vi "SendMsg.vi"(8 "error in (no error)":errorcluster, 11 "DataIn":T1={"MsgPageSelect"=enum."Action", "LogType"=enum."Manual", "Msg"="", "Time"=""}) -> (0 "error out":errorcluster)   [LabVIEW 2019, in "MsgShowAndLog.lvlib"]
uses:
  MsgShowAndLog.lvlib
  Ctrl/MsgDataInput.ctl
  Ctrl/MsgPageSelect.ctl
  Ctrl/LogType.ctl
  global/MsgQue.vi
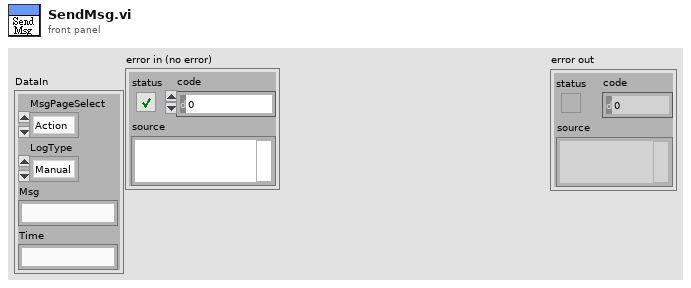
[diagram p1: front panel]
types:
  T1 = typedef "MsgDataInput.ctl" = cluster{"MsgPageSelect":T2, "LogType":T3, "Msg":string, "Time":string}
  T2 = typedef "MsgShowAndLog.lvlib/MsgPageSelect.ctl" = enum16{"System", "Comm", "IO", "Action", "Alarm"}
  T3 = typedef "MsgShowAndLog.lvlib/LogType.ctl" = enum16{"Auto", "Manual", "Handshake", "Error"}
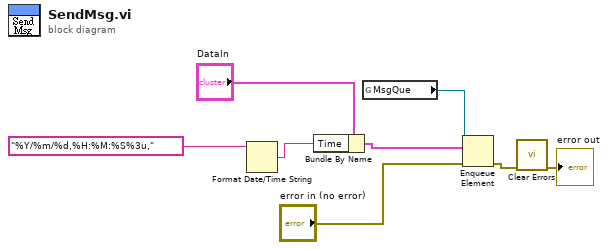
[diagram p0: block diagram]
diagram:
  n1 = Format Date/Time String(time format string (%c)="%Y/%m/%d,%H:%M:%S%3u,") -> (date/time string=w1:string)  [unwired: 2 in]
  n2 = Bundle By Name(cluster="DataIn", "Time"=w1) -> (w3:T1)
  n3 = global read "MsgQue.vi" "MsgQue"() -> (w8:refnum<queue>)
  n4 = Enqueue Element(queue=w8, element=w3, error in (no error)="error in (no error)") -> (error out=w6:errorcluster)  [unwired: 1 in, 2 out]
  n5 = call <vilib>:"Clear Errors.vi"("error in (no error)"=w6) -> ("error out"=→"error out":errorcluster)  [unwired: 5 in, 1 out]
